vi "X Running Sum.vi"(9 "Reset":bool, 11 "X Input":i16) -> (2 "X Running Sum":i16)   [LabVIEW 2010]
panel:
  # "Reset Sum to 0"
  # "Sum = Sum + X"
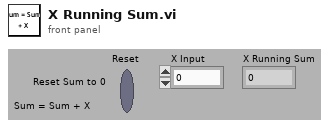
[diagram p1: front panel]
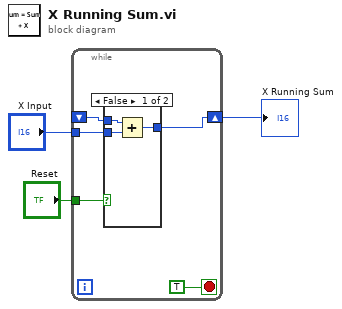
[diagram p0: block diagram]
diagram:
  n1 = while {
    shift-right: [w6] -> w1
    shift-left: _ -> [w7]
    tunnel: "X Input" -> [w8]
    tunnel: "Reset" -> [w5]
    stop <- TRUE stop-if-true
    n2 = case shown="False" w5 {
      tunnel: w8 -> [w11 w12]
      tunnel: w7 -> [w10 _]
      tunnel: [w9 w12] -> w6
      frame False {
        n3 = Add(x=w10, y=w11) -> (x+y=w9:i16)
      }
      frame True {
      }
    }
  }
  "X Running Sum" <- w1
